vi "oa_FIR Filter Based Sample Rate Conversion (Continuous) (N channels).vi"(7 "reset? (T)":bool=TRUE, 8 "FIR filter specifications":T2={"alias rejection (dB)"=120.0, "normalized bandwidth"=0.4536} {"normalized bandwidth" format="%.4f"; "alias rejection (dB)" format="%.2f"}, 9 "even angle position info":T1, 10 "dr":dbl=1.0 format="%.2p", 11 "even angle signals":cluster{"r0":dbl, "dr":dbl, "Y":dbl[]}[](array[cluster]) {"r0" format="%.2p"; "dr" format="%.2p"; "Y" format="%.2f"}) -> (0 "error out":errorcluster, 2 "out even angle position info out":T1, 3 "even angle signals out":cluster{"r0":dbl, "dr":dbl, "Y":dbl[]}[](array[cluster]) {"r0" format="%.2p"; "dr" format="%.2p"; "Y" format="%.2f"})   [LabVIEW 2017, in "SoundVib_OAUtility.lvlib"]
uses:
  <vilib>/addons/Sound and Vibration/Order Analysis/Utility/SoundVib_OAUtility.lvlib
  <vilib>/addons/Sound and Vibration/Order Analysis/Misc/OAT Position Info.ctl
  <vilib>/measure/maresamp.llb/Resample Waveform (continuous, t0 DBL).vi
  <vilib>/measure/maresamp.llb/Resample N Waveforms (continuous, t0 DBL).vi
  <vilib>/measure/NI_MAPro.lvlib
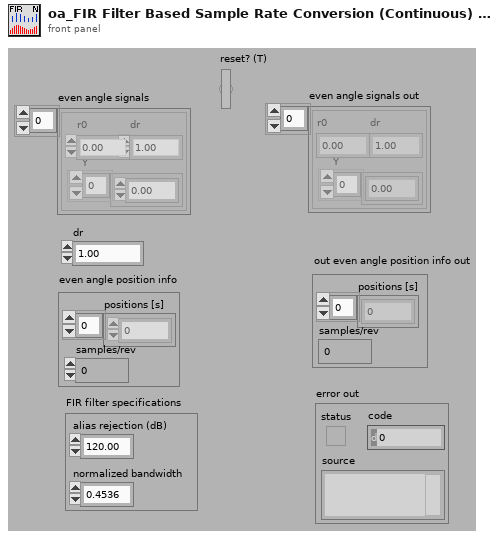
[diagram p1: front panel]
types:
  T1 = typedef "OAT Position Info.ctl" = cluster{"positions [s]":dbl[], "samples/rev":dbl}
  T2 = cluster{"alias rejection (dB)":dbl, "normalized bandwidth":dbl}
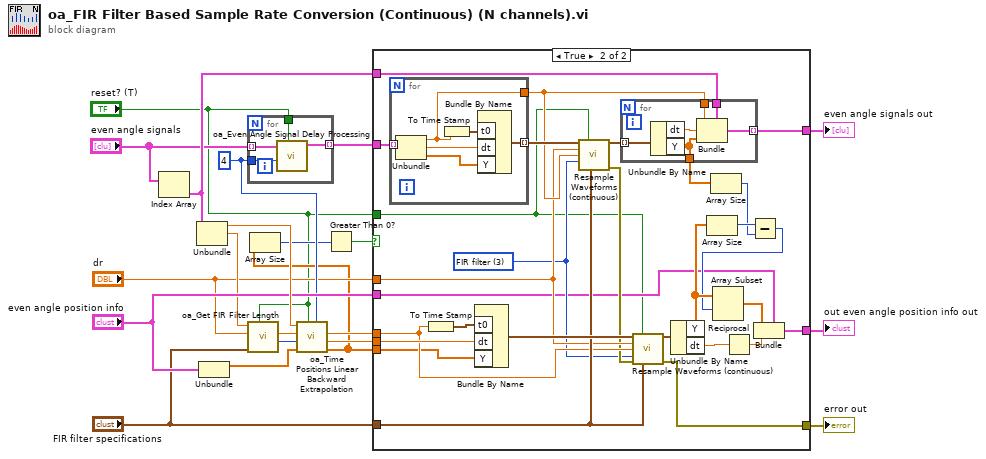
[diagram p0: block diagram]
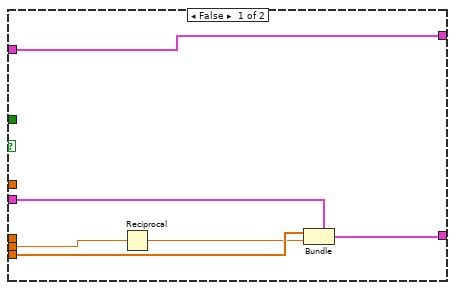
[diagram p2: hidden frame]
diagram:
  w15 = 4 ("number of points")
  n1 = Index Array(array="even angle signals") -> (element=w4:cluster{"r0":dbl, "dr":dbl, "Y":dbl[]})  [unwired: 1 in]
  n2 = Unbundle(w4) -> ("r0"=w20:dbl, "dr"=w14:dbl)  [unwired: 1 out]
  n3 = Unbundle("even angle position info") -> ("positions [s]"=w21:dbl[])  [unwired: 1 out]
  n4 = for {
    tunnel: [w25] -> w17 mode=indexing
    tunnel: w15 -> [w24]
    tunnel: "reset? (T)" -> [w23]
    tunnel: "even angle signals" -> [w22] mode=indexing
    n5 = call <vilib>:"oa_Even Angle Signal Delay Processing.vi"("reset? (T)"=w23, "number of points"=w24, "even angle signal in"=w22) -> ("buffered even angle signal"=w25:cluster{"r0":dbl, "dr":dbl, "Y":dbl[]})  [unwired: 8 in]
  }
  n6 = call <vilib>:"oa_Get FIR Filter Length.vi"("reset? (T)"="reset? (T)", "FIR filter specifications"="FIR filter specifications", "dr new"="dr", "dr old"=w14) -> ("filter length"=w13:i32, "dr old out"=w12:dbl)  [unwired: 6 in]
  n7 = call <vilib>:"oa_Time Positions Linear Backward Extrapolation.vi"("number of points"=w15, "reset? (T)"="reset? (T)", "positions [s]"=w21, "filter length"=w13, "dr"=w12, "r0"=w20) -> ("extraploated positions [s]"=w5:dbl[], "dr out"=w10:dbl, "new r0"=w9:dbl)  [unwired: 3 in]
  n8 = Array Size(array=w5) -> (size(s)=w8:i32)
  n9 = Greater Than 0?(x=w8) -> (x > 0?=w6:bool)
  n10 = case shown="True" w6 {
    tunnel: "reset? (T)" -> [_ w32]
    tunnel: "even angle position info" -> [w30 w33]
    tunnel: [w29 w54] -> w18
    tunnel: w17 -> [w31 w53]
    tunnel: "FIR filter specifications" -> [_ w51]
    tunnel: w4 -> [_ w49]
    tunnel: [w31 w47] -> w2
    tunnel: "dr" -> [_ w46]
    tunnel: w10 -> [w27 w45]
    tunnel: w9 -> [_ w44]
    tunnel: w5 -> [w28 w43]
    tunnel: [_ w40] -> w7
    frame False {
      n11 = Reciprocal(x=w27) -> (1/x=w26:dbl)
      n12 = Bundle(cluster=w30, "positions [s]"=w28, "samples/rev"=w26) -> (w29:T1)
    }
    frame True {
      w41 = u16 3 items=["coerce", "linear", "spline", "FIR filter"] ("interpolation mode")
      n13 = for {
        tunnel: w53 -> [w71] mode=indexing
        tunnel: [w67] -> w52 mode=indexing
        tunnel: [w66] -> w48
        n14 = Unbundle(w71) -> ("r0"=w66:dbl, "dr"=w69:dbl, "Y"=w70:dbl[])
        n15 = To Time Stamp(1:w66) -> (0:w68:timestamp)
        n16 = Bundle By Name("t0"=w68, "dt"=w69, "Y"=w70) -> (w67:waveform(dbl))  [unwired: 1 in]
      }
      n17 = To Time Stamp(1:w44) -> (0:w58:timestamp)
      n18 = Bundle By Name("t0"=w58, "dt"=w45, "Y"=w43) -> (w59:waveform(dbl))  [unwired: 1 in]
      n19 = call-poly <vilib>:"Resample Waveforms (continuous).vi"("waveforms in"=w52, "reset"=w32, "dt"=w46, "t0"=w48, "interpolation mode"=w41, "FIR filter specifications"=w51) -> ("resampled waveforms out"=w50:waveform(dbl)[], "error out"=w42:errorcluster)  [unwired: 5 in, 3 out]
      n20 = for {
        tunnel: w50 -> [w65] mode=indexing
        tunnel: w49 -> [w64]
        tunnel: w48 -> [w62]
        tunnel: [w61] -> w47 mode=indexing
        tunnel: [w60] -> w39
        n21 = Unbundle By Name(w65) -> ("dt"=w63:dbl, "Y"=w60:dbl[])
        n22 = Bundle(cluster=w64, "r0"=w62, "dr"=w63, "Y"=w60) -> (w61:cluster{"r0":dbl, "dr":dbl, "Y":dbl[]})
      }
      n23 = call-poly <vilib>:"Resample Waveforms (continuous).vi"("waveform in"=w59, "reset"=w32, "dt"=w46, "t0"=w44, "interpolation mode"=w41, "error in (no error)"=w42, "FIR filter specifications"=w51) -> ("resampled waveform out"=w57:waveform(dbl), "error out"=w40:errorcluster)  [unwired: 4 in, 3 out]
      n24 = Unbundle By Name(w57) -> ("Y"=w35:dbl[], "dt"=w56:dbl)
      n25 = Array Size(array=w35) -> (size(s)=w38:i32)
      n26 = Array Size(array=w39) -> (size(s)=w37:i32)
      n27 = Reciprocal(x=w56) -> (1/x=w55:dbl)
      n28 = Subtract(x=w38, y=w37) -> (x-y=w34:i32)
      n29 = Array Subset(array=w35, index=w34) -> (w36:dbl[])  [unwired: 1 in]
      n30 = Bundle(cluster=w33, "positions [s]"=w36, "samples/rev"=w55) -> (w54:T1)
    }
  }
  "out even angle position info out" <- w18
  "error out" <- w7
  "even angle signals out" <- w2
